vi "metadata grab based on inst ctrl states.vi"(6 "Sphere Indicator":T1=enum."Insulated Sphere", 7 "Analyzer Choice":T2, 8 "error in (no error)":errorcluster, 10 "Instrument Metadata":refnum<vi>, 11 "Instrument Control \nSwitches":T3) -> (0 "error out":errorcluster)   [LabVIEW 2014, in "Metadata.lvlib"]
uses:
  Metadata.lvlib
  controls/Instrument Control Switches.ctl
  controls/Analyzer Choice.ctl
  avantesSpectrometer/Acquisition/Sphere Indicator.ctl
  avantesSpectrometer/AvaSpec.lvlib
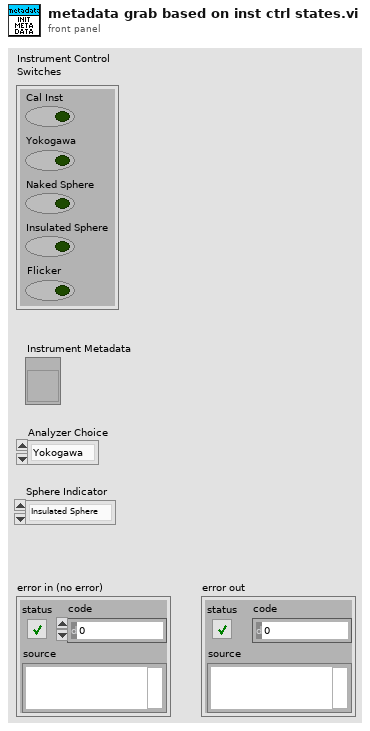
[diagram p1: front panel]
types:
  T1 = typedef "AvaSpec.lvlib/Sphere Indicator.ctl" = enum16{"Naked Sphere", "Insulated Sphere"}
  T2 = typedef "Analyzer Choice.ctl" = enum16{"Yokogawa", "Cal Inst"}
  T3 = typedef "Instrument Control Switches.ctl" = cluster{"Cal Inst":bool, "Yokogawa":bool, "Naked Sphere":bool, "Insulated Sphere":bool, "Flicker":bool}
  T4 = enum8{"Enabled", "Disabled", "Disabled and Grayed Out"}
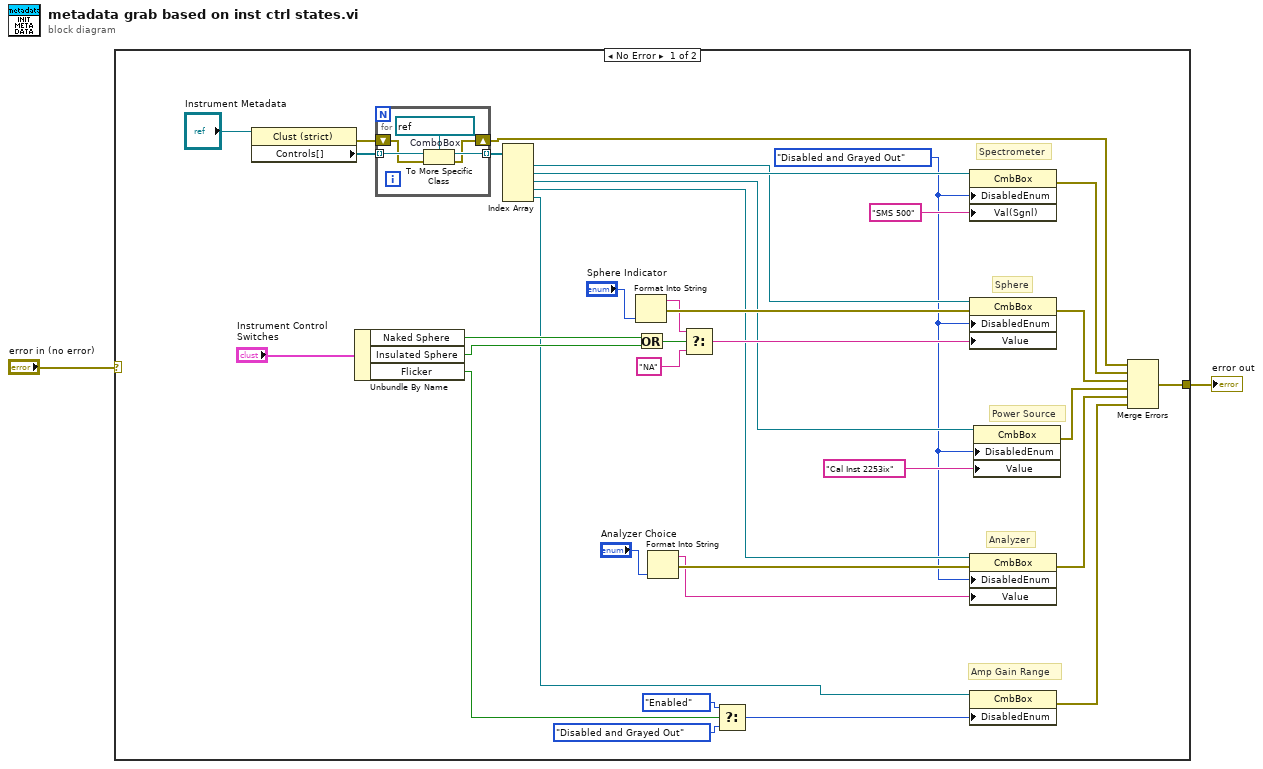
[diagram p0: block diagram]
diagram:
  n1 = case shown="No Error" "error in (no error)" {
    selector: "error in (no error)" -> [_ w43]
    tunnel: [w37 w43] -> w2
    frame No Error {
      w4 = T4."Disabled and Grayed Out" ("Disabled")
      # "Amp Gain Range"
      # "Analyzer"
      # "Power Source"
      # "Sphere"
      # "Spectrometer"
      n2 = property class="Clust (strict)"(reference="Instrument Metadata") -> (error out=w6:errorcluster, "Controls[]"=w13:refnum<vi>[])  [unwired: 1 in, 1 out]
      n3 = Unbundle By Name("Instrument Control \nSwitches") -> ("Naked Sphere"=w23:bool, "Insulated Sphere"=w24:bool, "Flicker"=w19:bool)
      n4 = for {
        tunnel: w13 -> [w41] mode=indexing
        tunnel: [w40] -> w12 mode=indexing
        shift-right: [w38] -> w5
        shift-left: w6 -> [w39]
        w42 = refnum<vi> refnum  # ComboBox
        n5 = To More Specific Class(target class=w42, reference=w41, error in=w39) -> (specific class reference=w40:refnum<vi>, error out=w38:errorcluster)
      }
      n6 = Index Array(array=w12) -> (element #1=w10:refnum<vi>, element #2=w11:refnum<vi>, element #3=w9:refnum<vi>, element #4=w8:refnum<vi>, element #5=w7:refnum<vi>)  [unwired: 5 in]
      n7 = Format Into String("Sphere Indicator") -> (resulting string=w26:string, error out=w30:errorcluster)  [unwired: 3 in]
      n8 = Or(x=w23, y=w24) -> (x .or. y?=w25:bool)
      n9 = Format Into String("Analyzer Choice") -> (resulting string=w22:string, error out=w31:errorcluster)  [unwired: 3 in]
      n10 = Select(t=w26, s=w25, f="NA") -> (s? t:f=w27:string)
      n11 = Select(t=T4."Enabled" ("Disabled"), s=w19, f=T4."Disabled and Grayed Out" ("Disabled")) -> (s? t:f=w18:T4)
      n12 = property class="CmbBox"(reference=w11, "DisabledEnum"=w4, "Val(Sgnl)"="SMS 500" ("Value")) -> (error out=w34:errorcluster)  [unwired: 1 in, 1 out]
      n13 = property class="CmbBox"(reference=w10, error in=w30, "DisabledEnum"=w4, "Value"=w27) -> (error out=w33:errorcluster)  [unwired: 1 out]
      n14 = property class="CmbBox"(reference=w8, error in=w31, "DisabledEnum"=w4, "Value"=w22) -> (error out=w35:errorcluster)  [unwired: 1 out]
      n15 = property class="CmbBox"(reference=w7, "DisabledEnum"=w18) -> (error out=w36:errorcluster)  [unwired: 1 in, 1 out]
      n16 = property class="CmbBox"(reference=w9, "DisabledEnum"=w4, "Value"="Cal Inst 2253ix") -> (error out=w32:errorcluster)  [unwired: 1 in, 1 out]
      n17 = Merge Errors(w5, w34, w33, w32, w35, w36) -> (w37:errorcluster)
    }
    frame Error {
    }
  }
  "error out" <- w2
